vi "Collect Actions.vi"(7 "Round":u32, 9 "Teams In":refnum<class "Team.lvclass">[](array[class]), 11 "Map in":refnum<class "Map.lvclass">) -> (1 "Teams":refnum<class "Team.lvclass">[](array[class]), 3 "Map out":refnum<class "Map.lvclass">)   [LabVIEW 2020, in "SquareBattle.lvlib" / "Map.lvclass"]
uses:
  Map.lvclass
  Team/Team.lvclass
  Map.lvclass/Map.ctl
  Position.ctl
  Run Result.ctl
  Action.ctl
  Direction.ctl
  Square/Square.lvclass
  Direction Offsets Const.vi
  SquareBattle.lvlib
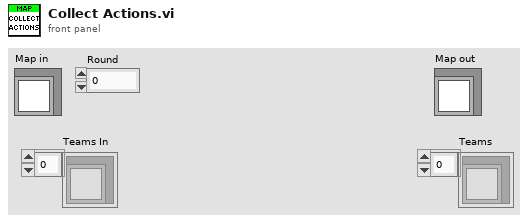
[diagram p1: front panel]
types:
  T1 = typedef "SquareBattle.lvlib/Position.ctl" = cluster{"Row":i32, "Col":i32}
  T2 = typedef "SquareBattle.lvlib/Run Result.ctl" = cluster{"Action":T3, "Direction":T4, "Replication":refnum<class "Square.lvclass">}
  T3 = typedef "SquareBattle.lvlib/Action.ctl" = enum16{"Wait", "Move", "Attack", "Replicate"}
  T4 = typedef "SquareBattle.lvlib/Direction.ctl" = enum16{"NW", "N", "NE", "E", "SE", "S", "SW", "W"}
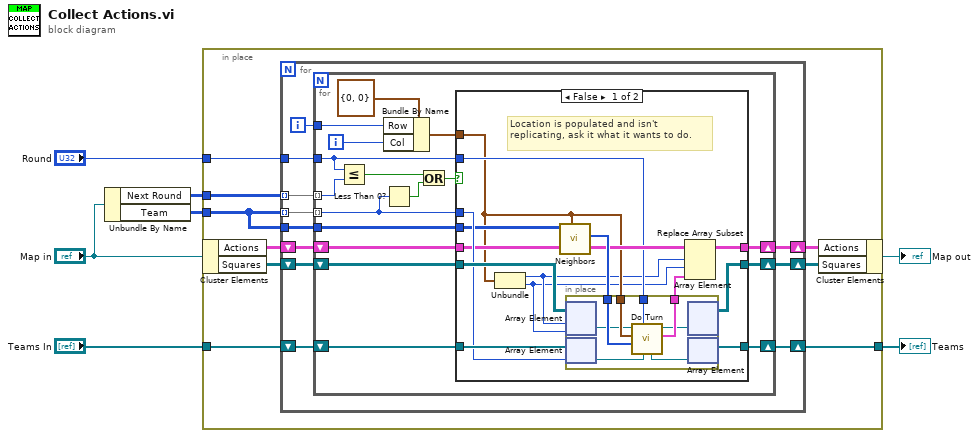
[diagram p0: block diagram]
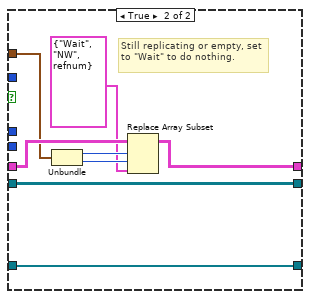
[diagram p2: hidden frame]
diagram:
  n1 = Unbundle By Name("Map in") -> ("Next Round"=w7:u32[][], "Team"=w6:i32[][])
  n2 = in-place {
    in-place-border: "Round" -> [w13]
    in-place-border: "Teams In" -> [w16]
    in-place-border: [w12] -> w1
    in-place-border: w7 -> [w11]
    in-place-border: w6 -> [w8]
    n3 = in-place-cluster #1("Map in") -> ("Actions"=w10:T2[][], "Squares"=w15:refnum<class "Square.lvclass">[][])
    n4 = for {
      shift-right: [w26] -> w12
      shift-left: w16 -> [w27]
      shift-right: [w24] -> w14
      shift-left: w15 -> [w25]
      shift-right: [w20] -> w9
      shift-left: w10 -> [w23]
      tunnel: w13 -> [w21]
      tunnel: w11 -> [w19] mode=indexing
      tunnel: w8 -> [w18] mode=indexing
      tunnel: w8 -> [w17]
      i -> [w22]
      n5 = for {
        shift-right: [w39] -> w26
        shift-left: w27 -> [w44]
        shift-right: [w40] -> w24
        shift-left: w25 -> [w43]
        shift-right: [w41] -> w20
        shift-left: w23 -> [w42]
        tunnel: w22 -> [w35]
        tunnel: w21 -> [w29]
        tunnel: w19 -> [w30] mode=indexing
        tunnel: w18 -> [w32] mode=indexing
        tunnel: w17 -> [w31]
        i -> [w34]
        n6 = Less Or Equal?(x=w29, y=w30) -> (x <= y?=w28:bool)
        n7 = Bundle By Name(cluster=T1 {"Row"=0, "Col"=0} ("Position"), "Row"=w35, "Col"=w34) -> (w33:T1)
        n8 = Less Than 0?(x=w32) -> (x < 0?=w38:bool)
        n9 = Or(x=w28, y=w38) -> (x .or. y?=w37:bool)
        n10 = case shown="False" w37 {
          tunnel: w44 -> [w57 w73]
          tunnel: w43 -> [w58 w74]
          tunnel: w42 -> [w53 w72]
          tunnel: [w51 w67] -> w41
          tunnel: [w50 w74] -> w40
          tunnel: [w54 w73] -> w39
          tunnel: w32 -> [w56 _]
          tunnel: w33 -> [w47 w69]
          tunnel: w31 -> [w49 _]
          tunnel: w29 -> [w48 _]
          frame False {
            # "Location is populated and isn't replicating, ask it what it wants to do."
            n11 = Unbundle(w47) -> ("Row"=w46:i32, "Col"=w45:i32)
            n12 = call "Neighbors.vi"("Position"=w47, "Team In"=w49) -> ("Neighbors"=w55:i32[])  [unwired: 8 in, 1 out]
            n13 = in-place {
              in-place-border: w48 -> [w66]
              in-place-border: w47 -> [w65]
              in-place-border: w55 -> [w64]
              in-place-border: [w61] -> w52
              n14 = in-place-array #2(w58, w46, w45) -> (w60:refnum<class "Square.lvclass">)
              n15 = in-place-array #3(w57, w56) -> (w63:refnum<class "Team.lvclass">)
              n16 = call "Do Turn.vi"("Team in"=w63, "Round Number"=w66, "Neighbors"=w64, "Position"=w65, "Square in"=w60) -> ("Run Result"=w61:T2, "Square out"=w59:refnum<class "Square.lvclass">, "Team out"=w62:refnum<class "Team.lvclass">)  [unwired: 4 in]
              n17 = in-place-array #2(w59) -> (w50:refnum<class "Square.lvclass">[][])  [unwired: 2 out]
              n18 = in-place-array #3(w62) -> (w54:refnum<class "Team.lvclass">[])  [unwired: 1 out]
            }
            n19 = Replace Array Subset(array=w53, new element=w52, index (row)=w46, index (col)=w45) -> (w51:T2[][])
          }
          frame True {
            # "Still replicating or empty, set to \"Wait\" to do nothing."
            n20 = Unbundle(w69) -> ("Row"=w71:i32, "Col"=w70:i32)
            n21 = Replace Array Subset(array=w72, new element=T2 {"Action"=enum."Wait", "Direction"=enum."NW", "Replication"=refnum} ("new element/subarray"), index (row)=w71, index (col)=w70) -> (w67:T2[][])
          }
        }
      }
    }
    n22 = in-place-cluster #1("Actions"=w9, "Squares"=w14) -> (→"Map out":refnum<class "Map.lvclass">)
  }
  "Teams" <- w1
